vi "meas_date.vi"() -> ()   [LabVIEW 2012]
panel:
  out "attempts":T1(array[cluster]) {"VCT measurment's date"."Temperature" format="%.2g st. C"; "VCT measurment's date"."time" format="%<%Mm %S%1us >t "; "VCT measurment's date"."Current" format="%.3g A"; "VCT measurment's date"."Voltage" format="%.3g V"}
  out "VCT measurment date":T2(array[cluster]) {"Temperature" format="%.2g st. C"; "time" format="%<%Mm %S%1us >t "; "Current" format="%.3g A"; "Voltage" format="%.3g V"}
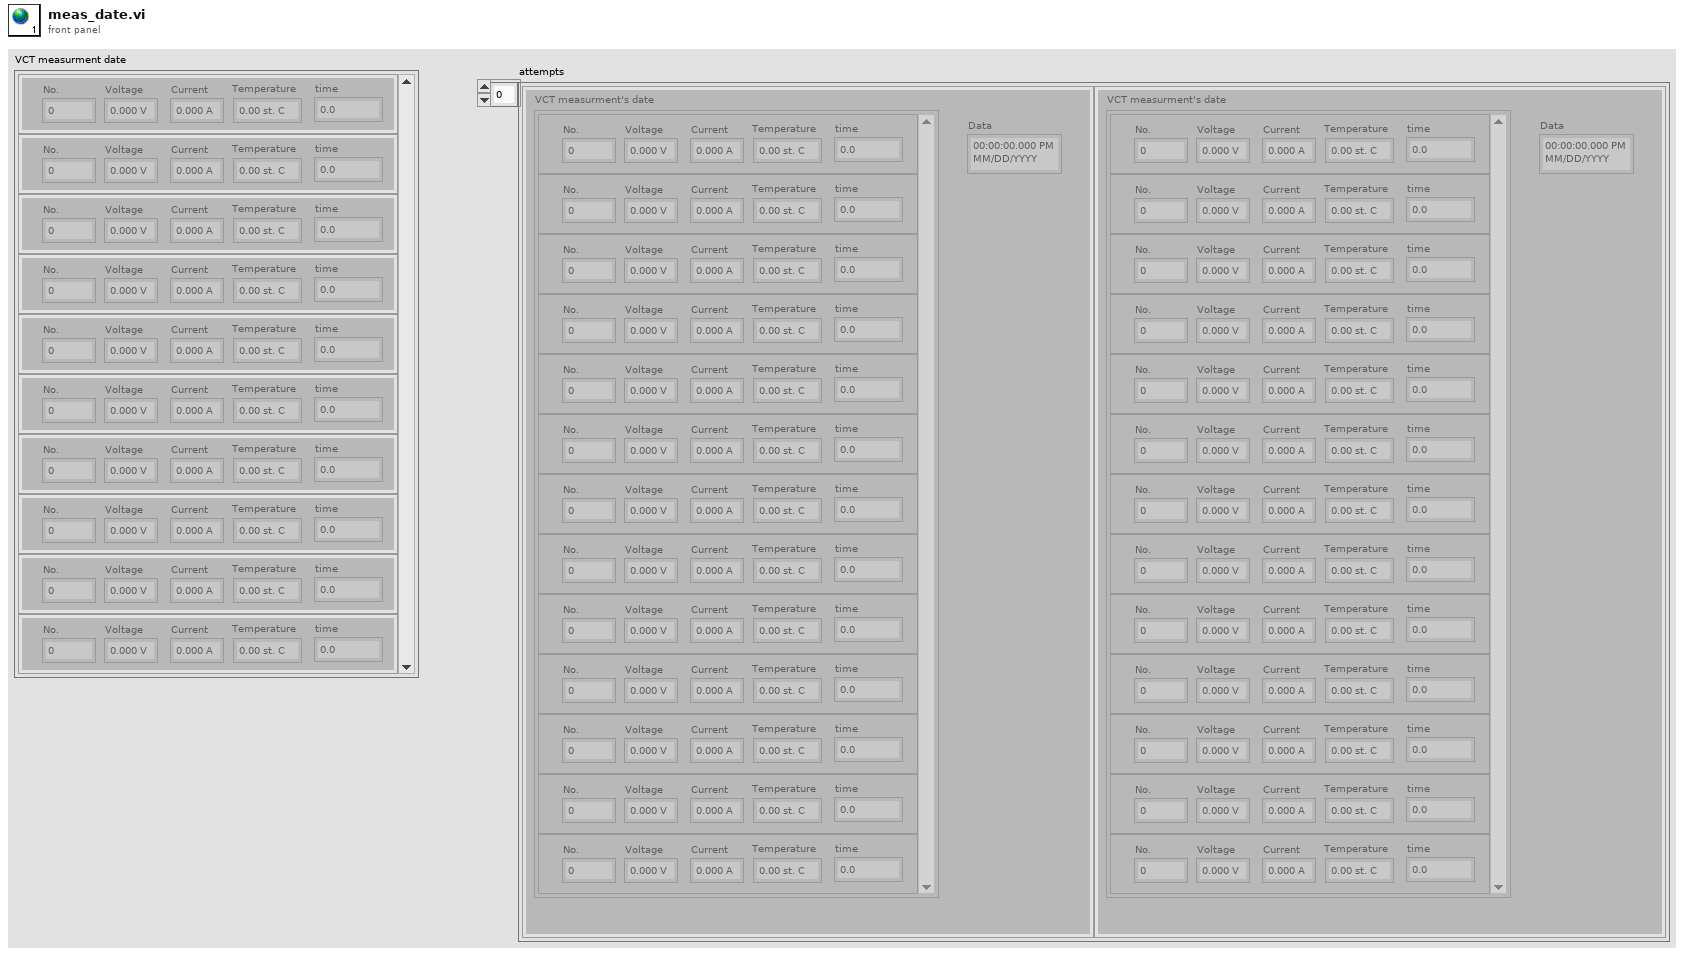
[diagram p1: front panel]
types:
  T1 = cluster{"VCT measurment's date":cluster{"No.":u64, "Voltage":dbl, "Current":dbl, "time":dbl, "Temperature":dbl}[], "Data":timestamp}[]
  T2 = cluster{"No.":u64, "Voltage":dbl, "Current":dbl, "time":dbl, "Temperature":dbl}[]
diagram:
